vi "Main.vi"() -> ()   [LabVIEW 2017]
doc: "The myRIO Project template acquires acceleration data from the onboard accelerometer and displays the changes of acceleration values in a waveform chart."
uses:
  Y Axis Motor Cluster.ctl
  X Axis Motor Cluster.ctl
  Coords Input Cluster.ctl
  Motor Status Enum.ctl
  Encoder Cluster.ctl
  <vilib>/myRIO/Common/Instrument Driver Framework/myRIO v1.0/Encoder/typedefs/Encoder Count Direction Enum.ctl
  Motion Type Def.ctl
  <vilib>/myRIO/Instrument Drivers/Onboard IO/PWM/typedefs/PWM Reference.ctl
  <vilib>/myRIO/Common/Instrument Driver Framework/Utilities/typedefs/myRIO Generic Hardware Reference.ctl
  <vilib>/myRIO/Common/Instrument Driver Framework/Utilities/typedefs/Hardware Version Enum.ctl
  <vilib>/myRIO/Common/Instrument Driver Framework/Utilities/typedefs/myRIO v1.0 Reference.ctl
  <vilib>/myRIO/Common/Instrument Driver Framework/Utilities/typedefs/Generic FPGA Reference.ctl
  <vilib>/myRIO/Common/Instrument Driver Framework/myRIO v1.0/PWM/typedefs/PWM Channels Enum.ctl
  <vilib>/myRIO/Instrument Drivers/Onboard IO/PWM/typedefs/PWM Configuration.ctl
  <vilib>/userdefined/High Color/nirio_resource_hc.ctl
  <vilib>/myRIO/Common/Instrument Driver Framework/Utilities/vis/Is FPGA Ref Available.vi
  <vilib>/myRIO/Common/Instrument Driver Framework/myRIO v1.0/PWM/vis/myRIO v1.1 Open PWM.vi
  <vilib>/myRIO/Instrument Drivers/Onboard IO/PWM/vis/Set Duty Cycle and Frequency.vi
  <vilib>/myRIO/Common/Instrument Driver Framework/Utilities/vis/Validate Channels.vi
  <vilib>/myRIO/Common/Instrument Driver Framework/myRIO v1.0/PWM/vis/myRIO v1.0 Reserve PWM.vi
  <vilib>/myRIO/Common/Instrument Driver Framework/myRIO v1.0/UART/vis/myRIO v1.0 Close UART.vi
  <vilib>/myRIO/Common/Instrument Driver Framework/myRIO v1.0/PWM/vis/myRIO v1.0 Build MUX Configuration PWM.vi
  <vilib>/myRIO/Common/Instrument Driver Framework/myRIO v1.0/Resource Manager/vis/myRIO v1.0 Reserve Channel List.vi
  <vilib>/myRIO/Common/Instrument Driver Framework/myRIO v1.0/Resource Manager/vis/myRIO v1.0 Create Configuration List.vi
  <vilib>/myRIO/Common/Instrument Driver Framework/myRIO v1.0/Resource Manager/vis/myRIO v1.0 Reserve Channel.vi
  <vilib>/myRIO/Common/Instrument Driver Framework/myRIO v1.0/Resource Manager/vis/myRIO v1.0 Unreserve Channel.vi
  <vilib>/myRIO/Common/Instrument Driver Framework/myRIO v1.0/Resource Manager/vis/myRIO v1.0 Build Mutex Name.vi
  <vilib>/addons/control/pid/pid.llb/PID Control Input Filter (DBL).vi
  <vilib>/addons/control/pid/pid.llb/PID (DBL).vi
  <vilib>/Utility/VariantDataType/GetNumericInfo.vi
  <vilib>/Utility/error.llb/Error Cluster From Error Code.vi
  <vilib>/myRIO/Common/Instrument Driver Framework/myRIO v1.0/myRIO v1.1 Open.vi
  <vilib>/myRIO/Common/Instrument Driver Framework/Utilities/vis/IO Manager.vi
  <vilib>/myRIO/Common/Instrument Driver Framework/Utilities/vis/Configuration Manager.vi
  <vilib>/myRIO/Common/Instrument Driver Framework/myRIO v1.0/Resource Manager/vis/myRIO v1.0 Configure IO.vi
  <vilib>/myRIO/Common/Instrument Driver Framework/myRIO v1.0/myRIO v1.0 Close.vi
  <vilib>/myRIO/Common/Instrument Driver Framework/myRIO v1.0/PWM/vis/myRIO v1.0 Write PWM.vi
  <vilib>/myRIO/Common/Instrument Driver Framework/Utilities/vis/FPGA Ref Manager.vi
  <vilib>/myRIO/Common/Instrument Driver Framework/myRIO v1.0/myRIO v1.0 Reset FPGA.vi
  <vilib>/myRIO/Common/Instrument Driver Framework/myRIO v1.0/IRQ/vis/myRIO v1.0 IRQ Info FGV.vi
  <vilib>/myRIO/Common/Instrument Driver Framework/myRIO v1.0/IRQ/vis/myRIO v1.0 Timer IRQ Info FGV.vi
  <vilib>/myRIO/Common/Instrument Driver Framework/myRIO v1.0/IRQ/vis/myRIO v1.0 ISR Agent.vi
  <vilib>/myRIO/Express VI/Onboard IO/PWM/PWM Express VI.xnode
  <vilib>/myRIO/Instrument Drivers/Onboard IO/PWM/vis/myRIO PWM Open.xnode
  <vilib>/myRIO/Instrument Drivers/Utilities/Utilities.lvlib
  <vilib>/myRIO/Instrument Drivers/Onboard IO/PWM/PWM.lvlib
  <vilib>/addons/control/pid/NI_PID_pid.lvlib
panel:
  out "Y Velocity":dbl[](graph)
  out "Motion Data":T1
  out "Converted\nPWM Duty%":dbl
  in  "X Axis PID Gains":T2={"proportional gain (Kc)"=1.0, "integral time (Ti, min)"=0.01, "derivative time (Td, min)"=0.0} {"derivative time (Td, min)" format="%.3f"; "integral time (Ti, min)" format="%.3f"; "proportional gain (Kc)" format="%.3f"}
  in  "Y Axis PID Gains":T2={"proportional gain (Kc)"=1.0, "integral time (Ti, min)"=0.01, "derivative time (Td, min)"=0.0} {"derivative time (Td, min)" format="%.3f"; "integral time (Ti, min)" format="%.4f"; "proportional gain (Kc)" format="%.3f"}
  out "Y Velocity overlaid":cluster{"Velocity Array":dbl[]}[](graph)
  out "Y Planned velocity":dbl[](graph)
  out "Completed?":bool
  out "Y freq + accel > max speed":bool
  out "Converted Decel":dbl
  out "Converted Accel":dbl
  out "Motion Profile":T3=enum."Triangular"
  out "Converted\nPWM Freq":dbl
  in  "Y Axis Setpoint":T4
  out "Encoder Output":T5
  out "X Axis state":T7
  out "Y Axis state":T7
  out "Loop Runtime (s)":dbl format="%.3f"
  in  "Coordinates Input":T8={"X-axis (mm)"=0.0, "Y-axis (mm)"=0.0, "X dist target\nthreshold (mm)"=0.0, "Y dist  target \nthreshold (mm)"=1.0} {"Y dist  target \nthreshold (mm)" min=0.0; "X dist target\nthreshold (mm)" min=0.0}
  out "Y Axis":T9(graph)
  out "X Axis":T9(graph)
  in  "X Axis Setpoint":T10
  out "X Axis Motor Params":T11
  out "Y Axis Motor Params":T12
  in  "stop":bool
  out "Total Runtime (s)":dbl format="%.2f"
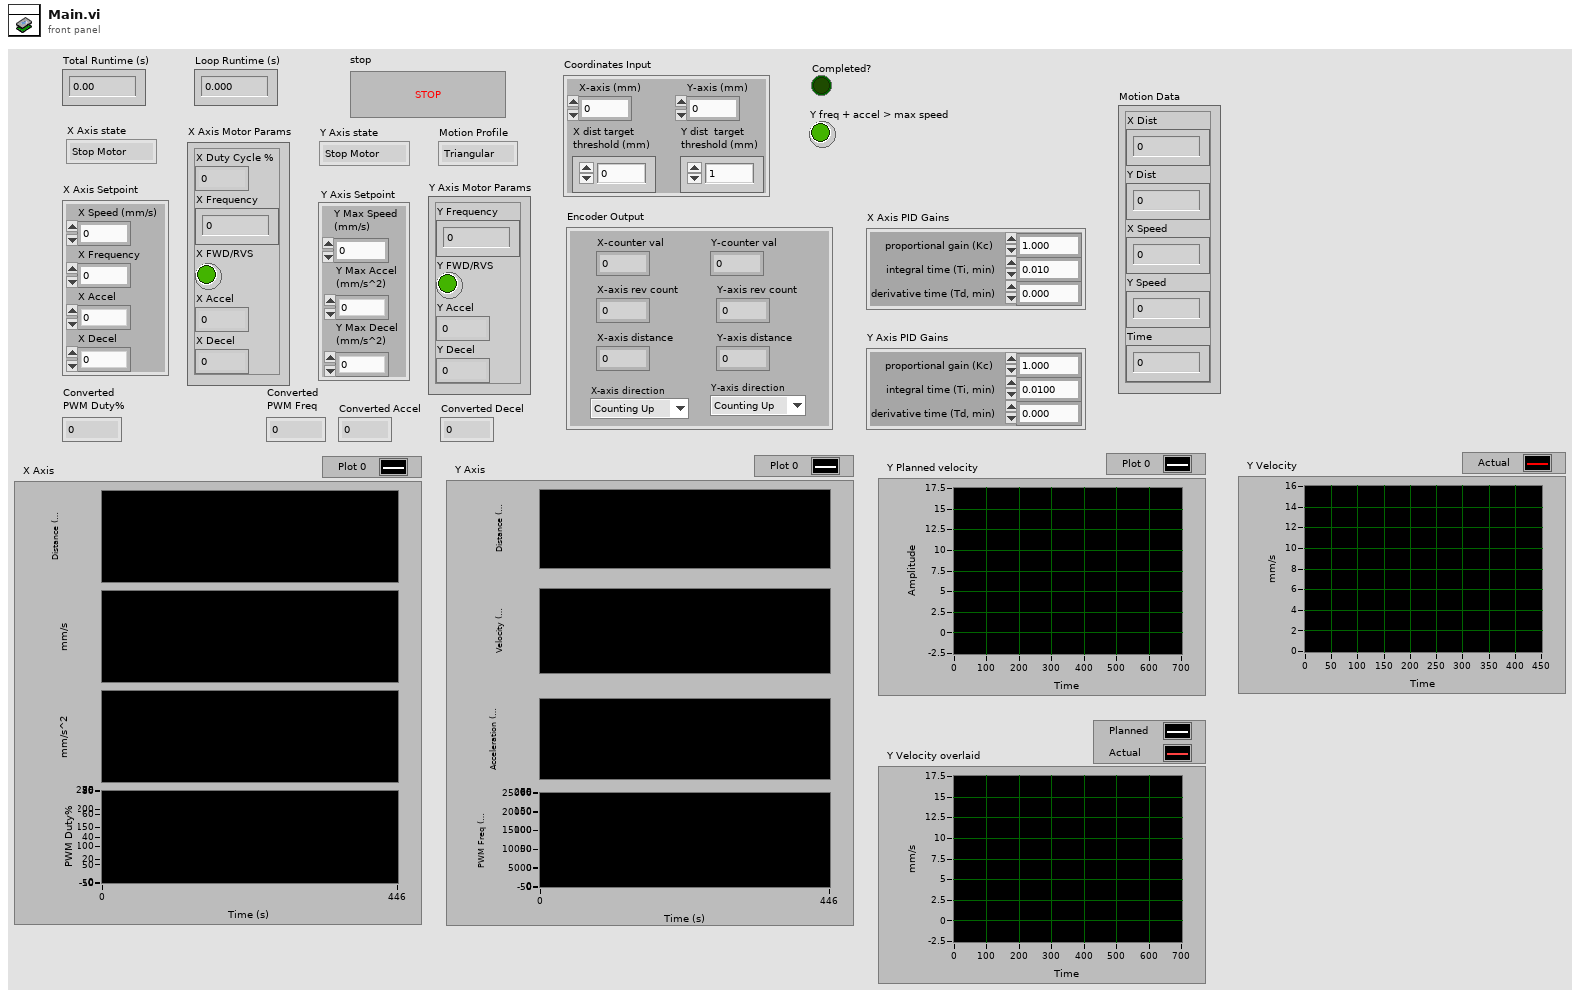
[diagram p1: front panel]
types:
  T1 = cluster{"X Dist":dbl, "Y Dist":dbl, "X Speed":dbl, "Y Speed":dbl, "Time":u32}
  T2 = cluster{"proportional gain (Kc)":dbl, "integral time (Ti, min)":dbl, "derivative time (Td, min)":dbl}
  T3 = typedef "Motion Type Def.ctl" = enum16{"Trapezodial", "Triangular"}
  T4 = cluster{"Y Max Speed \n(mm/s)":dbl, "Y Max Accel\n(mm/s^2)":dbl, "Y Max Decel \n(mm/s^2)":dbl}
  T5 = typedef "Encoder Cluster.ctl" = cluster{"Y-axis rev count":dbl, "Y-axis distance":dbl, "X-axis rev count":dbl, "X-axis distance":dbl, "Y-axis direction":T6, "X-axis direction":T6, "X-counter val":i32, "Y-counter val":i32}
  T6 = typedef "Encoder Count Direction Enum.ctl" = enum16{"Counting Up", "Counting Down"}
  T7 = typedef "Motor Status Enum.ctl" = enum16{"Stop Motor", "Read Inputs", "Steady Speed", "Accelerate", "Decelerate"}
  T8 = typedef "Coords Input Cluster.ctl" = cluster{"X-axis (mm)":dbl, "Y-axis (mm)":dbl, "X dist target\nthreshold (mm)":dbl, "Y dist  target \nthreshold (mm)":dbl}
  T9 = cluster{"X-axis distance":dbl, dbl, dbl, "X Frequency":dbl}
  T10 = cluster{"X Frequency":dbl, "X Accel":dbl, "X Decel":dbl, "X Speed (mm/s)":dbl}
  T11 = typedef "X Axis Motor Cluster.ctl" = cluster{"X Frequency":dbl, "X FWD/RVS":bool, "X Accel":dbl, "X Decel":dbl, "X Duty Cycle %":dbl}
  T12 = typedef "Y Axis Motor Cluster.ctl" = cluster{"Y Frequency":dbl, "Y FWD/RVS":bool, "Y Accel":dbl, "Y Decel":dbl}
  T13 = cluster{"Target Coords (mm)":dbl, "Current Coords (mm)":dbl, "Max Speed (mm/s)":dbl, "Max Accel (mm/s^2)":dbl, "Max Decel (mm/s^2)":dbl}
  T14 = cluster{" Distance target (mm)":dbl, "Max Accel (mm/s^2)":dbl, "Max Decel (mm/s^2)":dbl, "Velocity Limit (mm/s) ":dbl, "Time step (s)":dbl}
  T15 = enum16{"800", "1600", "3200", "6400", "12800", "25600"}
  T16 = cluster{"X-axis distance":dbl, dbl, dbl, "X Frequency":dbl}[]
  T17 = cluster{"Cruising Speed (mm/s)":dbl, "Crusing Time (s)":dbl, "Decel Time (s)":dbl, "Accel Time (s)":dbl, "Total Time (s)":dbl, "Accel Distance (mm)":dbl, "Decel Distance (mm)":dbl, "Crusing Distance (mm)":dbl}
  T18 = cluster{"X-axis distance":dbl, dbl, dbl, "X Duty Cycle %":dbl}
  T19 = cluster{"Y-axis distance":dbl, dbl, dbl, "Y Frequency":dbl}
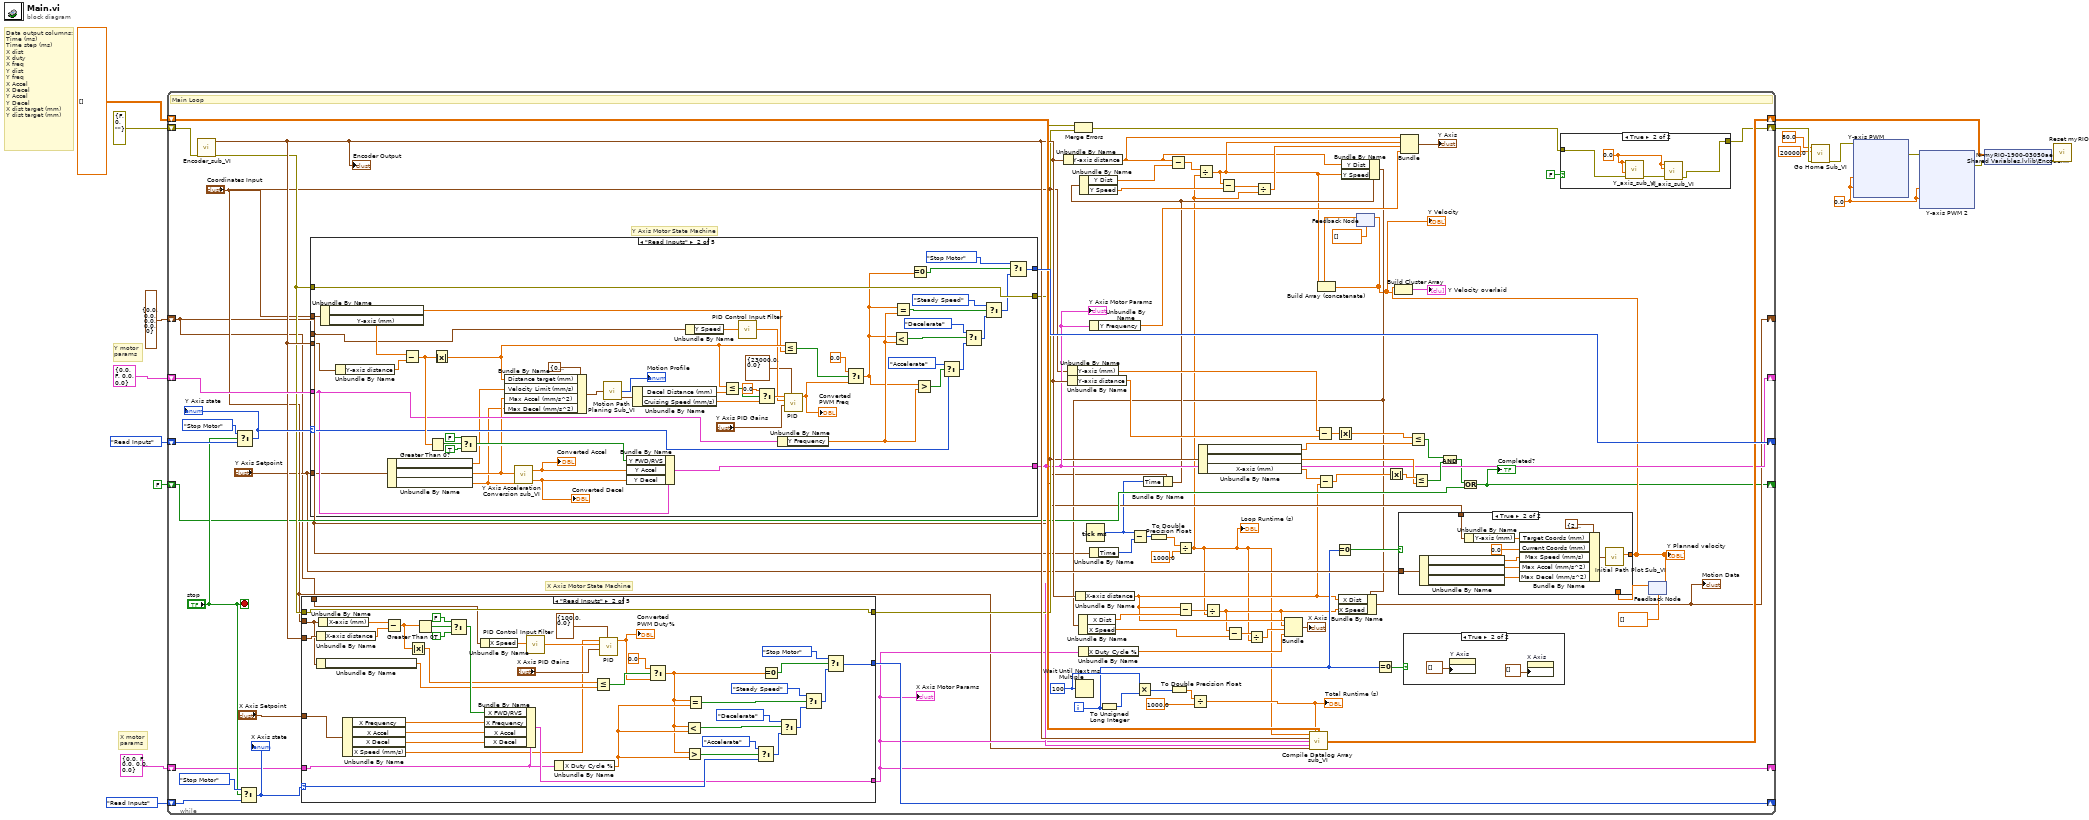
[diagram p0: block diagram]
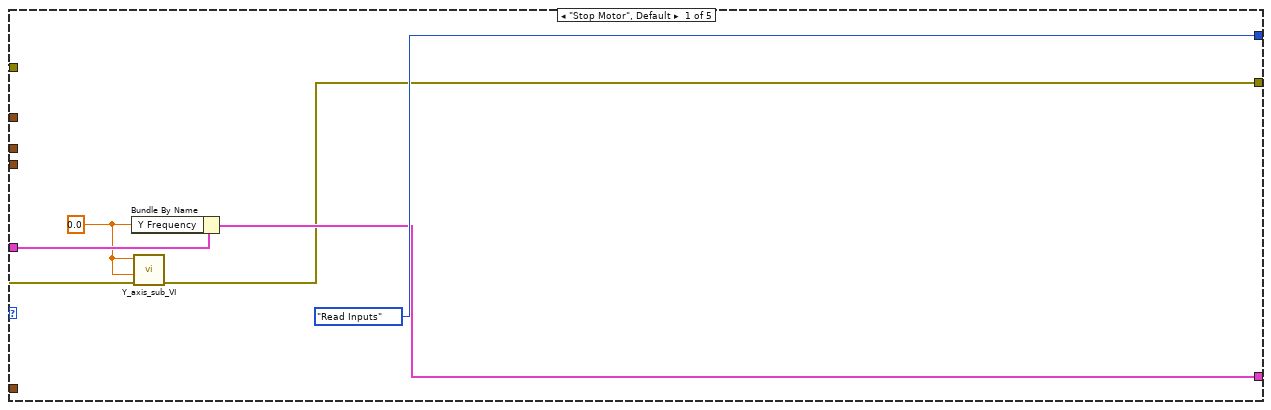
[diagram p4: hidden frame]
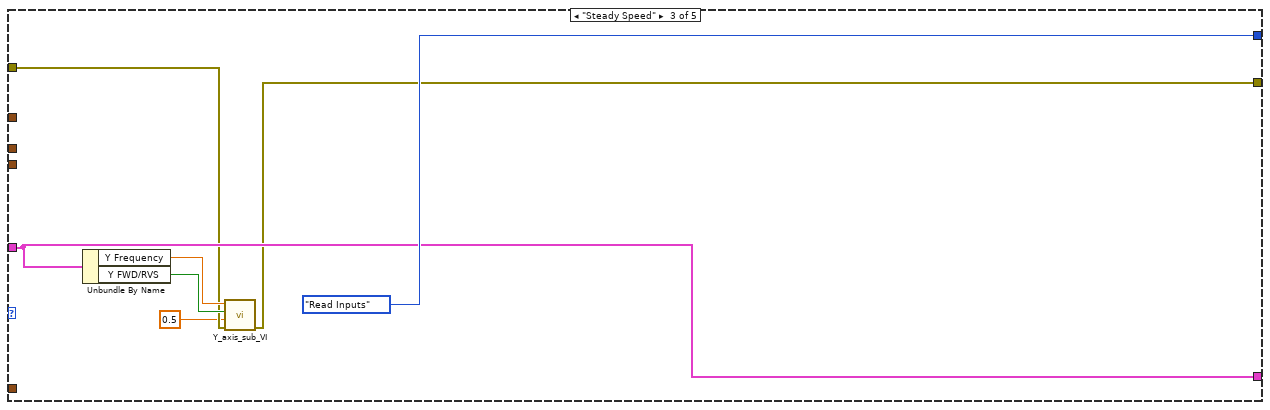
[diagram p5: hidden frame]
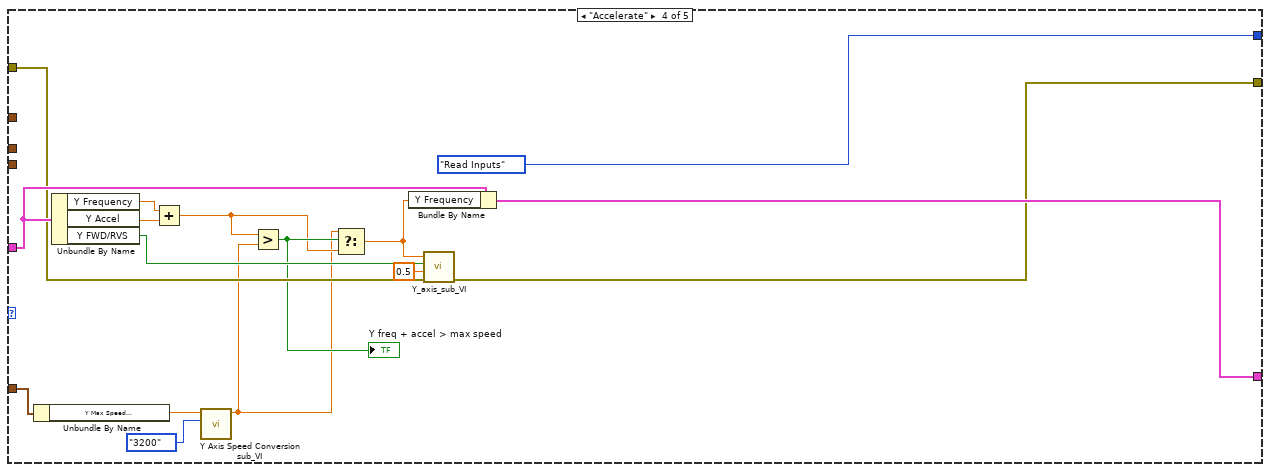
[diagram p6: hidden frame]
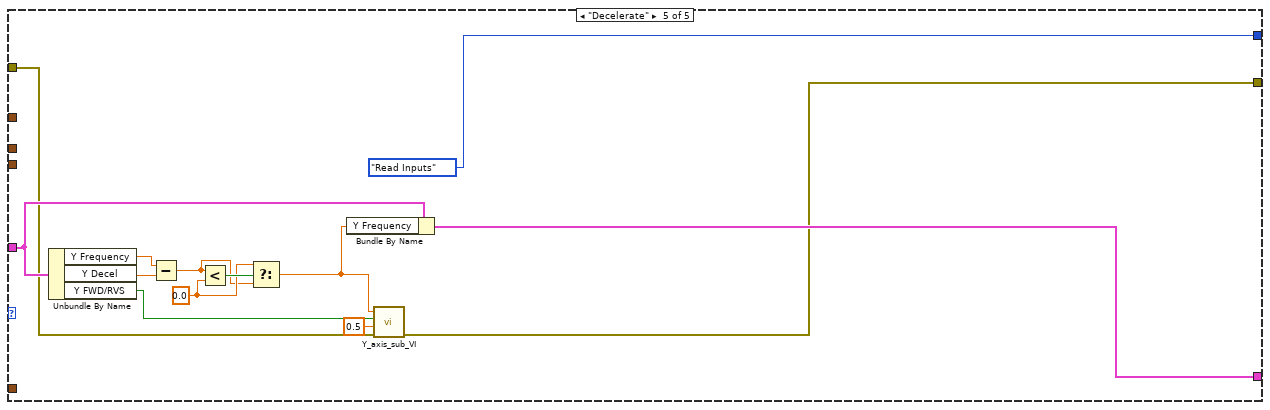
[diagram p7: hidden frame]
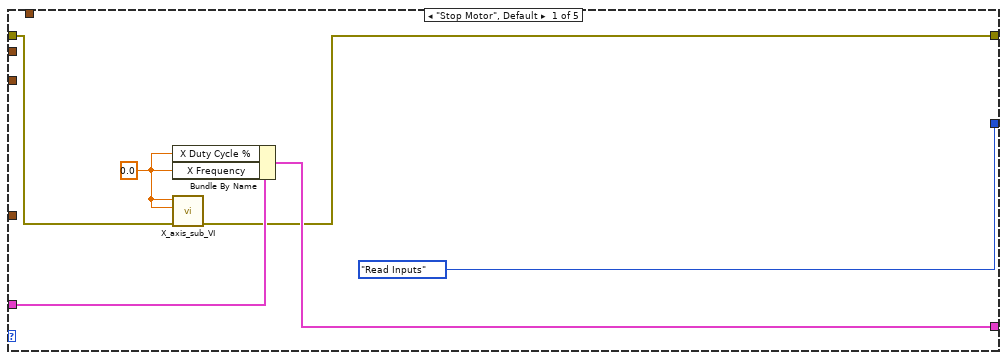
[diagram p9: hidden frame]
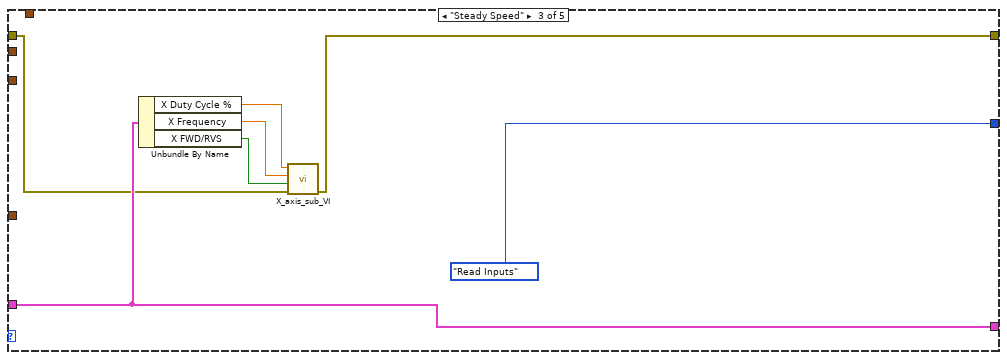
[diagram p10: hidden frame]
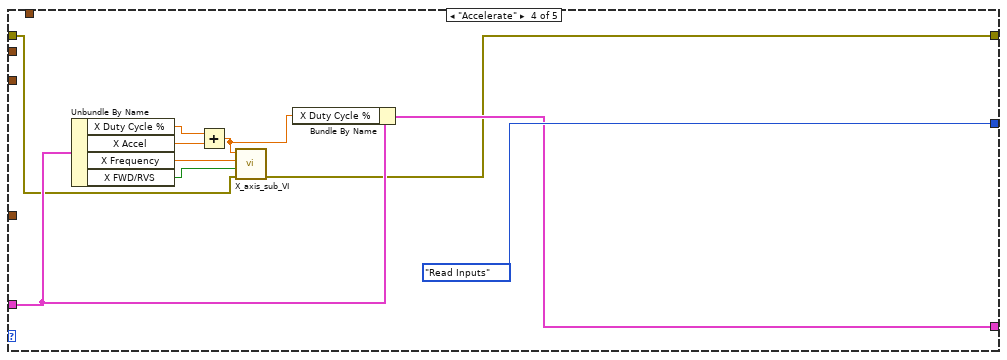
[diagram p11: hidden frame]
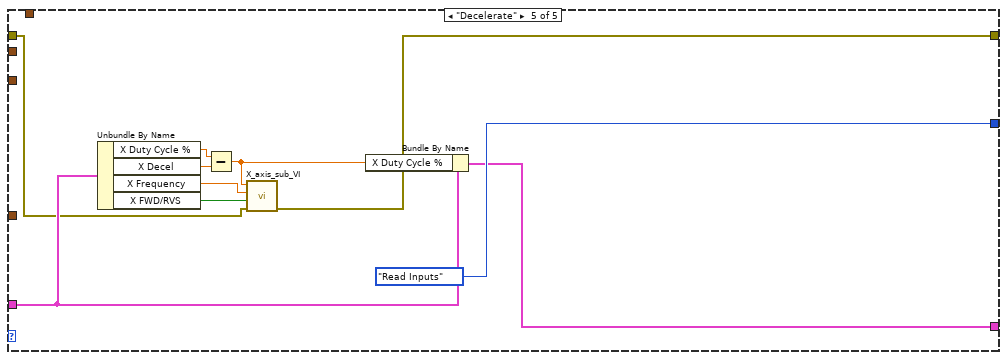
[diagram p12: hidden frame]
diagram:
  w2 = 0.0 ("Frequency [Hz]")
  # "X motor \nparams"
  # "Y motor \nparams"
  # "Data output columns:\nTime (ms)\nTime step (ms)\nX dist\nX duty\nX freq\nY dist\nY freq\nX Accel\nX Decel\nY Accel\nY Decel\nX dist target (mm)\nY dist target (mm)"
  n1 = while {
    shift-right: [w50] -> w9
    shift-left: errorcluster {"status"=FALSE, "code"=0, "source"=""} ("error in (no error)") -> [w101]
    shift-right: [w80] -> w10
    shift-left: dbl[][] [] -> [w81]
    shift-right: [w56] -> _
    shift-left: T12 {"Y Frequency"=0.0, "Y FWD/RVS"=FALSE, "Y Accel"=0.0, "Y Decel"=0.0} ("Y Axis Motor Params") -> [w100]
    shift-right: [w99] -> _
    shift-left: Motor_Status_Enum."Read Inputs" -> [w97]
    shift-right: [w91] -> _
    shift-left: Motor_Status_Enum."Read Inputs" -> [w93]
    shift-right: [w55] -> _
    shift-left: T11 {"X Frequency"=0.0, "X FWD/RVS"=FALSE, "X Accel"=0.0, "X Decel"=0.0, "X Duty Cycle %"=0.0} ("X Axis Motor Params") -> [w90]
    shift-right: [w19] -> _
    shift-left: FALSE -> [w53]
    shift-right: [w30] -> _
    shift-left: T1 {"X Dist"=0.0, "Y Dist"=0.0, "X Speed"=0.0, "Y Speed"=0.0, "Time"=0} ("Motion Data") -> [w25]
    i -> [w44]
    stop <- "stop" stop-if-true
    w85 = u32 100 ("milliseconds to wait")
    # "Y Axis Motor State Machine"
    # "X Axis Motor State Machine"
    # "Main Loop"
    n2 = call "Encoder_sub_VI.vi"("error in (no error)"=w101) -> ("error out"=w57:errorcluster, "Encoder Output"=w71:T5)  [unwired: 9 in]
    "Encoder Output" <- w71
    n3 = Select(t=Motor_Status_Enum."Stop Motor", s="stop", f=w97) -> (s? t:f=w98:T7)
    "Y Axis state" <- w98
    n4 = Select(t=Motor_Status_Enum."Stop Motor", s="stop", f=w93) -> (s? t:f=w94:T7)
    "X Axis state" <- w94
    n5 = case shown="\"Read Inputs\"" w94 {
      selector: w94 -> [_ w249 _ _ _]
      tunnel: [Motor_Status_Enum."Read Inputs" w232 Motor_Status_Enum."Read Inputs" Motor_Status_Enum."Read Inputs" Motor_Status_Enum."Read Inputs"] -> w91
      tunnel: [w216 w248 w265 w272 w282] -> w55
      tunnel: w90 -> [w217 w247 w265 w271 w281]
      tunnel: w57 -> [w215 w246 w263 w270 w280]
      tunnel: [w214 w246 w262 w269 w279] -> w58
      tunnel: w71 -> [_ w245 _ _ _]
      tunnel: "Coordinates Input" -> [_ w235 _ _ _]
      tunnel: w25 -> [_ w228 _ _ _]
      tunnel: "X Axis Setpoint" -> [_ w221 _ _ _]
      frame "Stop Motor", Default {
        w219 = 0.0 ("Y Frequency")
        n6 = Bundle By Name(cluster=w217, "X Duty Cycle %"=w219, "X Frequency"=w219) -> (w216:T11)
        n7 = call "X_axis_sub_VI.vi"("error in (no error)"=w215, "Frequency"=w219, "Duty Cycle %"=w219) -> ("error out"=w214:errorcluster)  [unwired: 8 in]
      }
      frame "Read Inputs" {
        n8 = Unbundle By Name(w245) -> ("X-axis distance"=w239:dbl)
        n9 = Unbundle By Name(w235) -> ("X dist target\nthreshold (mm)"=w234:dbl)
        n10 = Unbundle By Name(w235) -> ("X-axis (mm)"=w240:dbl)
        n11 = Unbundle By Name(w221) -> ("X Frequency"=w252:dbl, "X Accel"=w250:dbl, "X Decel"=w251:dbl, "X Speed (mm/s)"=w223:dbl)
        n12 = Subtract(x=w240, y=w239) -> (x-y=w237:dbl)
        n13 = Absolute Value(x=w237) -> (abs(x)=w236:dbl)
        n14 = Greater Than 0?(x=w237) -> (x > 0?=w243:bool)
        n15 = Select(t=FALSE, s=w243, f=TRUE) -> (s? t:f=w241:bool)
        n16 = Unbundle By Name(w228) -> ("X Speed"=w225:dbl)
        n17 = Bundle By Name(cluster=w247, "X FWD/RVS"=w241, "X Frequency"=w252, "X Accel"=w250, "X Decel"=w251) -> (w248:T11)
        n18 = call-poly <vilib>:"PID Control Input Filter.vi"("input"=w225) -> ("output"=w224:dbl)  [unwired: 4 in]
        n19 = Unbundle By Name(w247) -> ("X Duty Cycle %"=w260:dbl)
        n20 = Less Or Equal?(x=w236, y=w234) -> (x <= y?=w238:bool)
        n21 = call-poly <vilib>:"PID.vi"("output range"=cluster{"output high":dbl, "output low":dbl} {"output high"=100.0, "output low"=0.0}, "PID gains"="X Axis PID Gains", "process variable"=w224, "setpoint"=w223) -> ("output"=w220:dbl)  [unwired: 6 in, 1 out]
        "Converted\nPWM Duty%" <- w220
        n22 = Select(t=0.0, s=w238, f=w220) -> (s? t:f=w222:dbl)
        n23 = Less?(x=w222, y=w260) -> (x < y?=w255:bool)
        n24 = Greater?(x=w222, y=w260) -> (0:w253:bool)
        n25 = Equal?(x=w222, y=w260) -> (x = y?=w259:bool)
        n26 = Select(t=Motor_Status_Enum."Accelerate", s=w253, f=w249) -> (s? t:f=w257:T7)
        n27 = Equal To 0?(x=w222) -> (x = 0?=w229:bool)
        n28 = Select(t=Motor_Status_Enum."Decelerate", s=w255, f=w257) -> (s? t:f=w258:T7)
        n29 = Select(t=Motor_Status_Enum."Steady Speed", s=w259, f=w258) -> (s? t:f=w231:T7)
        n30 = Select(t=Motor_Status_Enum."Stop Motor", s=w229, f=w231) -> (s? t:f=w232:T7)
      }
      frame "Steady Speed" {
        n31 = Unbundle By Name(w265) -> ("X Duty Cycle %"=w267:dbl, "X Frequency"=w266:dbl, "X FWD/RVS"=w268:bool)
        n32 = call "X_axis_sub_VI.vi"("error in (no error)"=w263, "FWD/RVS"=w268, "Frequency"=w266, "Duty Cycle %"=w267) -> ("error out"=w262:errorcluster)  [unwired: 7 in]
      }
      frame "Accelerate" {
        n33 = Unbundle By Name(w271) -> ("X Duty Cycle %"=w274:dbl, "X Accel"=w275:dbl, "X Frequency"=w276:dbl, "X FWD/RVS"=w278:bool)
        n34 = Add(x=w274, y=w275) -> (x+y=w277:dbl)
        n35 = call "X_axis_sub_VI.vi"("error in (no error)"=w270, "FWD/RVS"=w278, "Frequency"=w276, "Duty Cycle %"=w277) -> ("error out"=w269:errorcluster)  [unwired: 7 in]
        n36 = Bundle By Name(cluster=w271, "X Duty Cycle %"=w277) -> (w272:T11)
      }
      frame "Decelerate" {
        n37 = Unbundle By Name(w281) -> ("X Duty Cycle %"=w284:dbl, "X Decel"=w285:dbl, "X Frequency"=w286:dbl, "X FWD/RVS"=w288:bool)
        n38 = Subtract(x=w284, y=w285) -> (x-y=w287:dbl)
        n39 = call "X_axis_sub_VI.vi"("error in (no error)"=w280, "FWD/RVS"=w288, "Frequency"=w286, "Duty Cycle %"=w287) -> ("error out"=w279:errorcluster)  [unwired: 7 in]
        n40 = Bundle By Name(cluster=w281, "X Duty Cycle %"=w287) -> (w282:T11)
      }
    }
    "X Axis Motor Params" <- w55
    n41 = case shown="\"Read Inputs\"" w98 {
      selector: w98 -> [_ w151 _ _ _]
      tunnel: w100 -> [w123 w147 w179 w195 w207]
      tunnel: [Motor_Status_Enum."Read Inputs" w125 Motor_Status_Enum."Read Inputs" Motor_Status_Enum."Read Inputs" Motor_Status_Enum."Read Inputs"] -> w99
      tunnel: [w121 w143 w179 w194 w208] -> w56
      tunnel: w57 -> [w119 w152 w178 w192 w205]
      tunnel: [w120 w152 w177 w191 w206] -> w59
      tunnel: w71 -> [_ w154 _ _ _]
      tunnel: "Coordinates Input" -> [_ w153 _ _ _]
      tunnel: "Y Axis Setpoint" -> [_ w144 _ w190 _]
      tunnel: w25 -> [_ w132 _ _ _]
      frame "Stop Motor", Default {
        w118 = 0.0 ("Y Frequency")
        n42 = Bundle By Name(cluster=w123, "Y Frequency"=w118) -> (w121:T12)
        n43 = call "Y_axis_sub_VI.vi"("error in (no error)"=w119, "Duty Cycle"=w118, "Frequency"=w118) -> ("error out"=w120:errorcluster)  [unwired: 8 in]
      }
      frame "Read Inputs" {
        n44 = Unbundle By Name(w153) -> ("Y dist  target \nthreshold (mm)"=w142:dbl, "Y-axis (mm)"=w133:dbl)
        n45 = Unbundle By Name(w154) -> ("Y-axis distance"=w141:dbl)
        n46 = Unbundle By Name(w144) -> ("Y Max Speed \n(mm/s)"=w140:dbl, "Y Max Accel\n(mm/s^2)"=w139:dbl, "Y Max Decel \n(mm/s^2)"=w138:dbl)
        n47 = Subtract(x=w133, y=w141) -> (x-y=w161:dbl)
        n48 = Greater Than 0?(x=w161) -> (x > 0?=w165:bool)
        n49 = Absolute Value(x=w161) -> (abs(x)=w145:dbl)
        n50 = Select(t=FALSE, s=w165, f=TRUE) -> (s? t:f=w166:bool)
        n51 = Bundle By Name(cluster=T14 {" Distance target (mm)"=0.0, "Max Accel (mm/s^2)"=0.0, "Max Decel (mm/s^2)"=0.0, "Velocity Limit (mm/s) "=0.0, "Time step (s)"=0.0} ("Motion Planning Inputs"), "Distance target (mm)"=w145, "Velocity Limit (mm/s)"=w140, "Max Accel (mm/s^2)"=w139, "Max Decel (mm/s^2)"=w138) -> (w163:T14)
        n52 = call "Y Axis Acceleration Conversion sub_VI.vi"("Deceleration (mm/s^2)"=w138, "Acceleration (mm/s^2)"=w139) -> ("Freq decrease per 0.1ms (Hz)"=w155:dbl, "Freq increase per 0.1ms (Hz)"=w156:dbl)
        "Converted Accel" <- w156
        "Converted Decel" <- w155
        n53 = call "Motion Path Planing Sub_VI.vi"("Motion Planning Inputs"=w163) -> ("Motion Profile"=→"Motion Profile":T3, "Motion Planning Outputs"=w137:T17)  [unwired: 4 in, 1 out]
        n54 = Bundle By Name(cluster=w147, "Y FWD/RVS"=w166, "Y Accel"=w156, "Y Decel"=w155) -> (w143:T12)
        n55 = Unbundle By Name(w137) -> ("Decel Distance (mm)"=w160:dbl, "Cruising Speed (mm/s)"=w149:dbl)
        n56 = Unbundle By Name(w132) -> ("Y Speed"=w131:dbl)
        n57 = Less Or Equal?(x=w145, y=w160) -> (x <= y?=w159:bool)
        n58 = call-poly <vilib>:"PID Control Input Filter.vi"("input"=w131) -> ("output"=w130:dbl)  [unwired: 4 in]
        n59 = Select(t=0.0, s=w159, f=w149) -> (s? t:f=w135:dbl)
        n60 = Unbundle By Name(w147) -> ("Y Frequency"=w148:dbl)
        n61 = Less Or Equal?(x=w145, y=w142) -> (x <= y?=w146:bool)
        n62 = call-poly <vilib>:"PID.vi"("output range"=cluster{"output high":dbl, "output low":dbl} {"output high"=23000.0, "output low"=0.0}, "PID gains"="Y Axis PID Gains", "process variable"=w130, "setpoint"=w135) -> ("output"=w136:dbl)  [unwired: 6 in, 1 out]
        "Converted\nPWM Freq" <- w136
        n63 = Select(t=0.0, s=w146, f=w136) -> (s? t:f=w128:dbl)
        n64 = Less?(x=w128, y=w148) -> (x < y?=w170:bool)
        n65 = Equal?(x=w128, y=w148) -> (x = y?=w173:bool)
        n66 = Equal To 0?(x=w128) -> (x = 0?=w127:bool)
        n67 = Greater?(x=w128, y=w148) -> (0:w150:bool)
        n68 = Select(t=Motor_Status_Enum."Accelerate", s=w150, f=w151) -> (s? t:f=w172:T7)
        n69 = Select(t=Motor_Status_Enum."Decelerate", s=w170, f=w172) -> (s? t:f=w174:T7)
        n70 = Select(t=Motor_Status_Enum."Steady Speed", s=w173, f=w174) -> (s? t:f=w126:T7)
        n71 = Select(t=Motor_Status_Enum."Stop Motor", s=w127, f=w126) -> (s? t:f=w125:T7)
      }
      frame "Steady Speed" {
        n72 = Unbundle By Name(w179) -> ("Y Frequency"=w181:dbl, "Y FWD/RVS"=w182:bool)
        n73 = call "Y_axis_sub_VI.vi"("error in (no error)"=w178, "Duty Cycle"=0.5, "FWD/RVS"=w182, "Frequency"=w181) -> ("error out"=w177:errorcluster)  [unwired: 7 in]
      }
      frame "Accelerate" {
        n74 = Unbundle By Name(w190) -> ("Y Max Speed \n(mm/s)"=w185:dbl)
        n75 = Unbundle By Name(w195) -> ("Y Frequency"=w197:dbl, "Y Accel"=w198:dbl, "Y FWD/RVS"=w193:bool)
        n76 = Add(x=w197, y=w198) -> (x+y=w188:dbl)
        n77 = call "Y Axis Speed Conversion sub_VI.vi"("Microsteps per Rev"=T15."3200", "Setpoint\nSpeed (mm/s)"=w185) -> ("PWM Frequency"=w184:dbl)  [unwired: 9 in]
        n78 = Greater?(x=w188, y=w184) -> (0:w189:bool)
        "Y freq + accel > max speed" <- w189
        n79 = Select(t=w184, s=w189, f=w188) -> (s? t:f=w187:dbl)
        n80 = Bundle By Name(cluster=w195, "Y Frequency"=w187) -> (w194:T12)
        n81 = call "Y_axis_sub_VI.vi"("error in (no error)"=w192, "Duty Cycle"=0.5, "FWD/RVS"=w193, "Frequency"=w187) -> ("error out"=w191:errorcluster)  [unwired: 7 in]
      }
      frame "Decelerate" {
        w202 = 0.0 ("y")
        n82 = Unbundle By Name(w207) -> ("Y Frequency"=w211:dbl, "Y Decel"=w210:dbl, "Y FWD/RVS"=w204:bool)
        n83 = Subtract(x=w211, y=w210) -> (x-y=w201:dbl)
        n84 = Less?(x=w201, y=w202) -> (x < y?=w203:bool)
        n85 = Select(t=w202, s=w203, f=w201) -> (s? t:f=w200:dbl)
        n86 = Bundle By Name(cluster=w207, "Y Frequency"=w200) -> (w208:T12)
        n87 = call "Y_axis_sub_VI.vi"("error in (no error)"=w205, "Duty Cycle"=0.5, "FWD/RVS"=w204, "Frequency"=w200) -> ("error out"=w206:errorcluster)  [unwired: 7 in]
      }
    }
    "Y Axis Motor Params" <- w56
    n88 = Unbundle By Name(w71) -> ("Y-axis distance"=w23:dbl)
    n89 = Unbundle By Name("Coordinates Input") -> ("Y-axis (mm)"=w49:dbl)
    n90 = Unbundle By Name(w71) -> ("Y-axis distance"=w48:dbl)
    n91 = Merge Errors(w59, w58) -> (w51:errorcluster)
    n92 = Wait Until Next ms Multiple(millisecond multiple=w85) -> ()  [unwired: 1 out]
    n93 = Unbundle By Name(w71) -> ("X-axis distance"=w28:dbl)
    n94 = Unbundle By Name(w55) -> ("X Duty Cycle %"=w78:dbl)
    n95 = Tick Count (ms)() -> (millisecond timer value=w21:u32)
    n96 = Unbundle By Name(w56) -> ("Y Frequency"=w69:dbl)
    n97 = Unbundle By Name(w25) -> ("Time"=w37:u32)
    n98 = To Unsigned Long Integer(number=w44) -> (unsigned 32bit integer=w84:u32)
    n99 = Subtract(x=w21, y=w37) -> (x-y=w36:u32)
    n100 = Multiply(x=w85, y=w84) -> (x*y=w83:u32)
    n101 = Bundle By Name(cluster=w25, "Time"=w21) -> (w34:T1)
    n102 = Unbundle By Name(w34) -> ("Y Dist"=w35:dbl, "Y Speed"=w32:dbl)
    n103 = To Double Precision Float(number=w36) -> (double precision float=w86:dbl)
    n104 = Subtract(x=w23, y=w35) -> (x-y=w77:dbl)
    n105 = To Double Precision Float(number=w83) -> (double precision float=w82:dbl)
    n106 = Divide(x=w86, y=1000.0) -> (x/y=w22:dbl)
    "Loop Runtime (s)" <- w22
    n107 = Divide(x=w82, y=1000.0) -> (x/y=w79:dbl)
    "Total Runtime (s)" <- w79
    n108 = Divide(x=w77, y=w22) -> (x/y=w33:dbl)
    n109 = Unbundle By Name("Coordinates Input") -> ("Y dist  target \nthreshold (mm)"=w65:dbl, "X dist target\nthreshold (mm)"=w62:dbl, "X-axis (mm)"=w61:dbl)
    n110 = Subtract(x=w33, y=w32) -> (x-y=w76:dbl)
    n111 = Divide(x=w76, y=w22) -> (x/y=w70:dbl)
    n112 = call "Compile Datalog Array sub_VI.vi"("Loop Runtime (s)"=w22, "Total Runtime (s)"=w79, "Initialised Array"=w81, "Encoder Output"=w71, "X Axis Motor Params"=w55, "Y Axis Motor Params"=w56, "Coordinates Input"="Coordinates Input") -> ("Data Array"=w80:dbl[][])  [unwired: 8 in]
    n113 = Subtract(x=w49, y=w48) -> (x-y=w68:dbl)
    n114 = Subtract(x=w61, y=w28) -> (x-y=w64:dbl)
    n115 = Equal To 0?(x=w44) -> (x = 0?=w45:bool)
    n116 = Absolute Value(x=w68) -> (abs(x)=w67:dbl)
    n117 = Bundle By Name(cluster=w34, "Y Dist"=w23, "Y Speed"=w33) -> (w31:T1)
    n118 = Unbundle By Name(w31) -> ("X Dist"=w29:dbl, "X Speed"=w27:dbl)
    n119 = Subtract(x=w28, y=w29) -> (x-y=w75:dbl)
    n120 = Divide(x=w75, y=w22) -> (x/y=w26:dbl)
    n121 = Subtract(x=w26, y=w27) -> (x-y=w74:dbl)
    n122 = Divide(x=w74, y=w22) -> (x/y=w73:dbl)
    n123 = Bundle("X-axis distance"=w28, w26, w73, "X Duty Cycle %"=w78) -> (→"X Axis":T18)  [unwired: 1 in]
    n124 = Bundle By Name(cluster=w31, "X Dist"=w28, "X Speed"=w26) -> (w30:T1)
    "Motion Data" <- w30
    n125 = feedback #1(dbl[] []) -> (w41:dbl[])
    n126 = Build Array (concatenate)(w41, w33) -> (w20:dbl[])
    "Y Velocity" <- w20
    n127 = feedback-in #1(w20) -> ()
    n128 = Equal To 0?(x=w44) -> (x = 0?=w52:bool)
    n129 = Absolute Value(x=w64) -> (abs(x)=w63:dbl)
    n130 = Bundle("Y-axis distance"=w23, w33, w70, "Y Frequency"=w69) -> (→"Y Axis":T19)  [unwired: 1 in]
    n131 = case shown="True" w52 {
      frame False {
      }
      frame True {
        n132 = property on="Y Axis" class="WFChart (strict)"("History Data"=T16 []) -> ()  [unwired: 2 in, 2 out]
        n133 = property on="X Axis" class="WFChart (strict)"("History Data"=T16 []) -> ()  [unwired: 2 in, 2 out]
      }
    }
    n134 = Less Or Equal?(x=w67, y=w65) -> (x <= y?=w66:bool)
    n135 = Less Or Equal?(x=w63, y=w62) -> (x <= y?=w60:bool)
    n136 = And(x=w66, y=w60) -> (x .and. y?=w54:bool)
    n137 = Or(x=w54, y=w53) -> (x .or. y?=w19:bool)
    "Completed?" <- w19
    n138 = case shown="True" FALSE {
      tunnel: w51 -> [w113 w117]
      tunnel: [w113 w115] -> w50
      frame False {
      }
      frame True {
        w114 = 0.0 ("Frequency [Hz]")
        n139 = call "Y_axis_sub_VI.vi"("error in (no error)"=w117, "Duty Cycle"=w114, "Frequency"=w114) -> ("error out"=w116:errorcluster)  [unwired: 8 in]
        n140 = call "X_axis_sub_VI.vi"("error in (no error)"=w116, "Frequency"=w114, "Duty Cycle %"=w114) -> ("error out"=w115:errorcluster)  [unwired: 8 in]
      }
    }
    n141 = feedback #2(dbl[] [] ("Velocity Array")) -> (w43:dbl[])
    n142 = case shown="True" w45 {
      tunnel: "Coordinates Input" -> [_ w110]
      tunnel: "Y Axis Setpoint" -> [_ w107]
      tunnel: [w102 w103] -> w38
      tunnel: w43 -> [w102 _]
      frame False {
      }
      frame True {
        n143 = Unbundle By Name(w107) -> ("Y Max Speed \n(mm/s)"=w106:dbl, "Y Max Accel\n(mm/s^2)"=w105:dbl, "Y Max Decel \n(mm/s^2)"=w104:dbl)
        n144 = Unbundle By Name(w110) -> ("Y-axis (mm)"=w109:dbl)
        n145 = Bundle By Name(cluster=T13 {"Target Coords (mm)"=200.0, "Current Coords (mm)"=0.0, "Max Speed (mm/s)"=15.0, "Max Accel (mm/s^2)"=10.0, "Max Decel (mm/s^2)"=5.0} ("Motion Inputs"), "Target Coords (mm)"=w109, "Current Coords (mm)"=0.0, "Max Speed (mm/s)"=w106, "Max Accel (mm/s^2)"=w105, "Max Decel (mm/s^2)"=w104) -> (w112:T13)
        n146 = call "Initial Path Plot Sub_VI.vi"("Motion Inputs"=w112) -> ("Velocity Array"=w103:dbl[])  [unwired: 4 in, 6 out]
      }
    }
    "Y Planned velocity" <- w38
    n147 = Build Cluster Array(w38, w20) -> (→"Y Velocity overlaid":cluster{"Velocity Array":dbl[]}[])
    n148 = feedback-in #2(w38) -> ()
  }
  n149 = call "Go Home Sub_VI.vi"("error in (no error)"=w9, "Homing Freq"=20000.0, "Homing Duty %"=80.0) -> ("error out"=w8:errorcluster)  [unwired: 7 in, 1 out]
  n150 = xnode "Y-axis PWM"("Duty Cycle"=w2, "Frequency [Hz]"=w2, "error in (no error)"=w8) -> ("error out"=w14:errorcluster)
  n151 = xnode "Y-axis PWM 2"("Duty Cycle"=w2, "Frequency [Hz]"=w2, "error in (no error)"=w14) -> ("error out"=w13:errorcluster)
  n152 = shared-variable "NI-myRIO-1900-03050ae4\\Shared Variables.lvlib\\Encoder Data"(w10, error in=w13) -> (error out=w15:errorcluster)
  n153 = call <vilib>:"Reset myRIO.vi"("error in (no error)"=w15) -> ()  [unwired: 10 in, 1 out]
